vi "getSweepResults.vi"(8 "error in (no error)":errorcluster, 11 "Instrument.LockinAPI in":refnum<class "Instrument.LockinAPI.lvclass">) -> (0 "error out":errorcluster, 1 "Y Results":waveform(dbl)[](array[waveform]), 2 "X results":waveform(dbl)[](array[waveform]), 3 "Instrument.LockinAPI out":refnum<class "Instrument.LockinAPI.lvclass">)   [LabVIEW 2019, in "Instrument.LockinAPI.lvclass"]
doc: "API to get the results of lockin calculation.\n\nIf address=\"\", this API reads from localhost\nIf address is remote lockin, you need to add this computer to allowed whitelist on the lockin computer you are trying to access."
uses:
  Instrument.LockinAPI.lvclass
  C:/Users/patrick/Documents/GitHub/Instrument-Framework/lvsrc/Instrument/Instrument.lvclass
  Typedefs/API/LockinAPI.Commands--Enum.ctl
  31f3b684-3642-40cf-9e33-c0a48a6f90f4.vi
  31f3b684-3642-40cf-9e33-c0a48a6f90f4.vi/a3965658-0840-44e0-9e7d-b087dece7a9f.vi
  31f3b684-3642-40cf-9e33-c0a48a6f90f4.vi/a3965658-0840-44e0-9e7d-b087dece7a9f.vi/29f9d78b-5ea3-41c4-9def-440a54a2c915.vi
  31f3b684-3642-40cf-9e33-c0a48a6f90f4.vi/a3965658-0840-44e0-9e7d-b087dece7a9f.vi/29f9d78b-5ea3-41c4-9def-440a54a2c915.vi/5a303641-6742-4458-9979-7a1f89b46af3.vi
  31f3b684-3642-40cf-9e33-c0a48a6f90f4.vi/a3965658-0840-44e0-9e7d-b087dece7a9f.vi/29f9d78b-5ea3-41c4-9def-440a54a2c915.vi/15cafa2c-18d1-41a6-9ec7-6632f25168cf.vi
  Instrument/Protected/Validate API method.vi
  Instrument/Private/Get RC Connection Status.vi
  Instrument/API/Send and Receive.vi
  <vilib>/Utility/Data Type/Get Type Information.vi
  <vilib>/JDP Science/JSONtext/JSON text to Variant.vi
  <vilib>/JDP Science/JSONtext/LVClass Serializer/JSONtext LVClass Serializer.lvclass
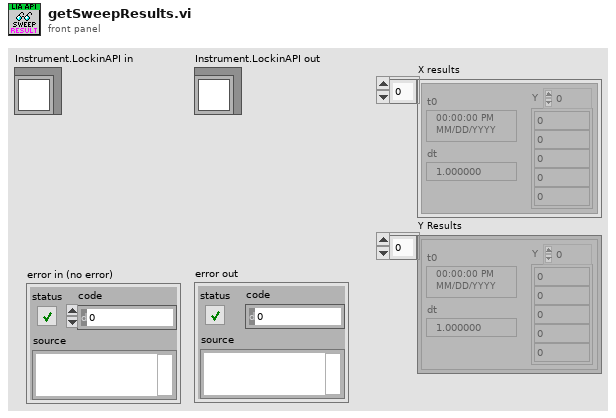
[diagram p1: front panel]
types:
  T1 = typedef "Instrument.LockinAPI.lvclass/LockinAPI.Commands--Enum.ctl" = enum16{"setAI", "setAO", "setAO_Amplitude", "setAO_DC", "setAO_Frequency", "setAO_Phase", "setAO_Function", "setAO_I+", "setREF", "setREF_Frequency", "setREF_Phase", "setREF_TC", "setREF_Roll-Off", "setDAQ", "setSampling", "setOffset", "setState", "getState", "getAO", "getAI", "getResults", "getSampling", "getAOconfig", "getREFconfig", "setInputGain", "setOutputGain", "getInputGain", "getOutputGain", "setSamplingMode", "getSamplingMode", "setSweep", "setSweepTime", "setSweepTable", "getStatus", "getSweepResults", "getSweepWaveforms", "startSweep", "stopSweep", "setAUX", "getAUX"}
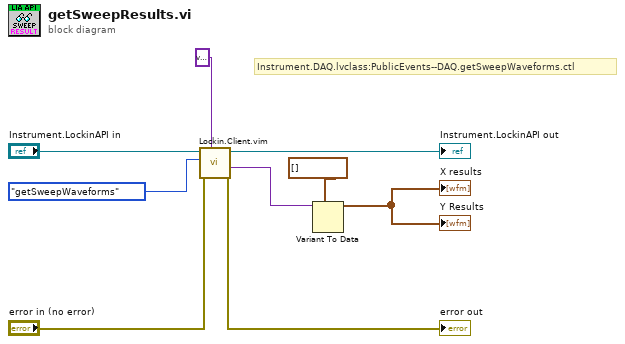
[diagram p0: block diagram]
diagram:
  # "Instrument.DAQ.lvclass:PublicEvents--DAQ.getSweepWaveforms.ctl"
  n1 = call "Lockin.Client.vim"("Data Out type"=variant, "error in (no error)"="error in (no error)", "Command"=LockinAPI.Commands--Enum."getSweepWaveforms", "Instrument.LockinAPI in"="Instrument.LockinAPI in") -> ("error out"=→"error out":errorcluster, "Data out"=w3:variant, "Instrument.LockinAPI out"=→"Instrument.LockinAPI out":refnum<class "Instrument.LockinAPI.lvclass">)  [unwired: 5 in]
  n2 = Variant To Data(type=waveform(dbl)[] [] ("X results"), Variant=w3) -> (data=→"X results" →"Y Results":waveform(dbl)[])  [unwired: 1 in, 1 out]
